vi "graph indicator.vi"() -> ()   [LabVIEW 2016]
panel:
  out "data":dynamicdata(graph)
  in  "Stop":bool
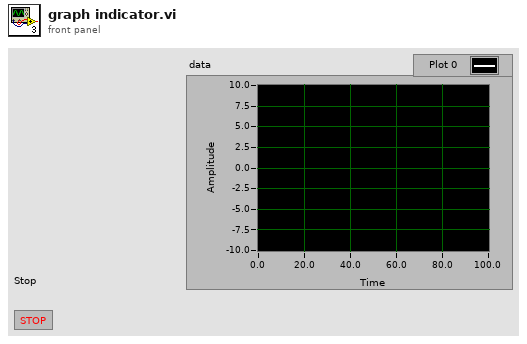
[diagram p1: front panel]
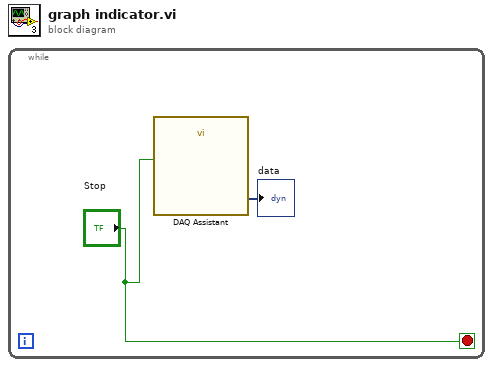
[diagram p0: block diagram]
diagram:
  n1 = while {
    stop <- "Stop" stop-if-true
    n2 = call "DAQ Assistant"("stop (T)"="Stop") -> ("data"=→"data":dynamicdata)  [unwired: 16 in, 2 out]
  }
